vi "Trata CMD PDA.vi"(4 "Comando":string="DEC MOTOR MOVER=12 34 56.7") -> (1 "String Enviado":string)   [LabVIEW 2018]
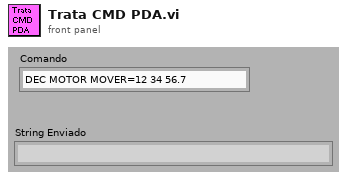
[diagram p1: front panel]
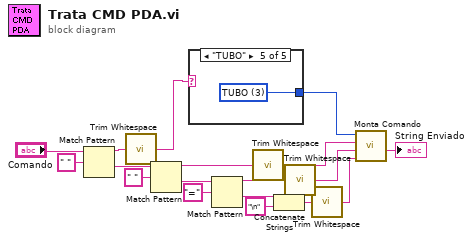
[diagram p0: block diagram]
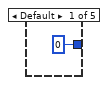
[diagram p2: hidden frame]
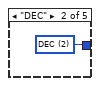
[diagram p3: hidden frame]
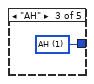
[diagram p4: hidden frame]
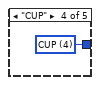
[diagram p5: hidden frame]
diagram:
  n1 = Match Pattern(string="Comando", regular expression=" ") -> (before substring=w10:string, after substring=w14:string)  [unwired: 1 in, 2 out]
  n2 = call <vilib>:"Trim Whitespace.vi"("string"=w10) -> ("trimmed string"=w4:string)  [unwired: 1 in]
  n3 = Match Pattern(string=w14, regular expression=" ") -> (before substring=w12:string, after substring=w13:string)  [unwired: 1 in, 2 out]
  n4 = case shown="\"TUBO\"" w4 {
    tunnel: [u16 0 ("Controlador") w20 w21 w22 w23] -> w9
    frame Default {
    }
    frame "DEC" {
      w20 = u16 2 items=["ZERO", "AH", "DEC", "TUBO", "CUP"] ("Controlador")
    }
    frame "AH" {
      w21 = u16 1 items=["ZERO", "AH", "DEC", "TUBO", "CUP"] ("Controlador")
    }
    frame "CUP" {
      w22 = u16 4 items=["ZERO", "AH", "DEC", "TUBO", "CUP"] ("Controlador")
    }
    frame "TUBO" {
      w23 = u16 3 items=["ZERO", "AH", "DEC", "TUBO", "CUP"] ("Controlador")
    }
  }
  n5 = Match Pattern(string=w13, regular expression="=") -> (before substring=w11:string, after substring=w8:string)  [unwired: 1 in, 2 out]
  n6 = call <vilib>:"Trim Whitespace.vi"("string"=w12) -> ("trimmed string"=w3:string)  [unwired: 1 in]
  n7 = Concatenate Strings(w8, "\n" ("string")) -> (w7:string)
  n8 = call <vilib>:"Trim Whitespace.vi"("string"=w11) -> ("trimmed string"=w2:string)  [unwired: 1 in]
  n9 = call <vilib>:"Trim Whitespace.vi"("string"=w7) -> ("trimmed string"=w1:string)  [unwired: 1 in]
  n10 = call "Monta Comando.vi"("Set Point"=w1, "Comando"=w2, "Dispositivo"=w3, "Controlador"=w9) -> ("String Enviado"=→"String Enviado":string)  [unwired: 1 in, 4 out]
